vi "SUB_Read_specifFile_anyFolder.vi"(2 "name or relative path":string, 3 "Base path":string) -> (0 "error out":errorcluster, 1 "text":string)   [LabVIEW 2011]
panel:
  out "path":path
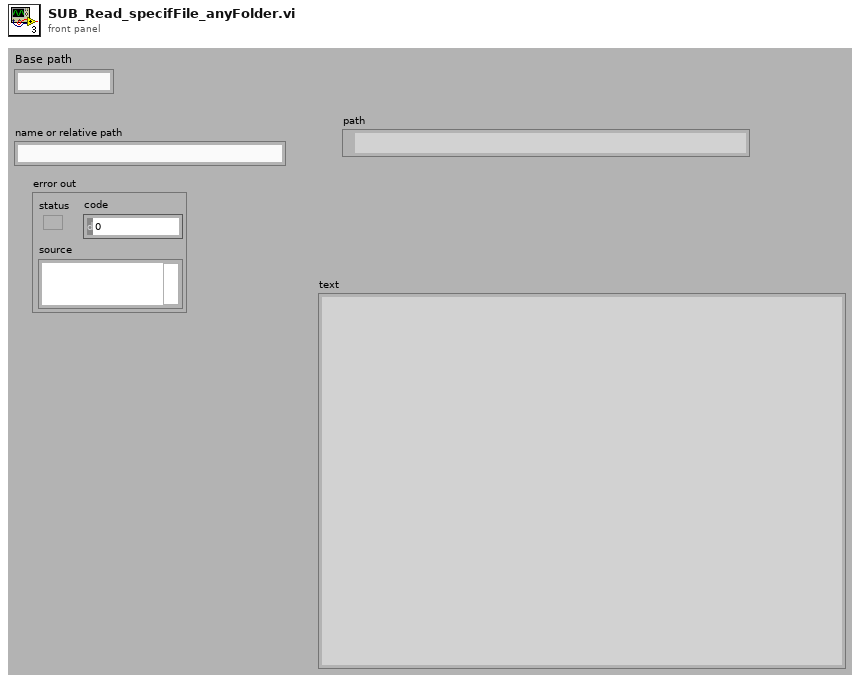
[diagram p1: front panel]
types:
  T1 = enum16{"open", "replace", "create", "open or create", "replace or create", "replace or create with confirmation"}
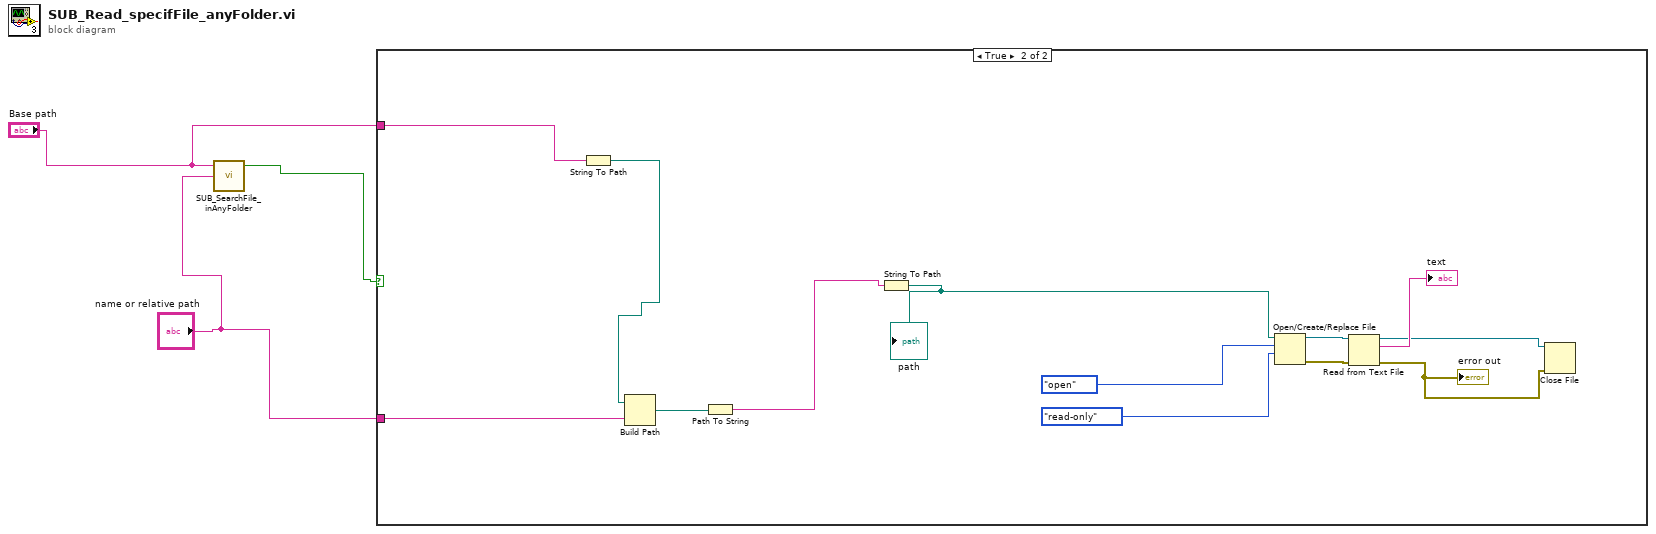
[diagram p0: block diagram]
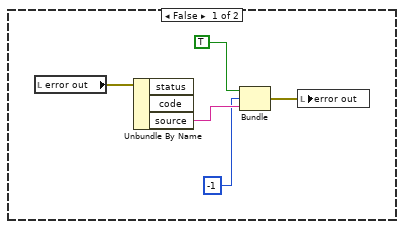
[diagram p2: hidden frame]
diagram:
  n1 = call "SUB_SearchFile_inAnyFolder.vi"("Search Filename in Folder"="name or relative path", "Base path"="Base path") -> ("File Existing True/Flase"=w1:bool)  [unwired: 1 in, 2 out]
  n2 = case shown="True" w1 {
    tunnel: "name or relative path" -> [_ w11]
    tunnel: "Base path" -> [_ w9]
    frame False {
      n3 = local read "error out"() -> (w8:errorcluster)
      n4 = Unbundle By Name(w8) -> ("source"=w7:string)  [unwired: 2 out]
      n5 = Bundle(TRUE, -1, "source"=w7) -> (w4:cluster{bool, i32, "source":string})  [unwired: 1 in]
      n6 = local write "error out"(w4) -> ()
    }
    frame True {
      n7 = String To Path(string=w9) -> (path=w10:path)
      n8 = Build Path(base path=w10, name or relative path=w11) -> (appended path=w13:path)
      n9 = Path To String(path=w13) -> (string=w12:string)
      n10 = String To Path(string=w12) -> (path=w16:path)
      "path" <- w16
      n11 = Open/Create/Replace File(file path (use dialog)=w16, operation (0:open)=T1."open", access (0:read/write)=enum16{"read/write", "read-only", "write-only"}."read-only") -> (refnum out=w19:refnum<file>, error out=w18:errorcluster)  [unwired: 3 in, 1 out]
      n12 = Read from Text File(file (use dialog)=w19, error in=w18) -> (refnum out=w15:refnum<file>, text=→"text":string, error out=w14:errorcluster)  [unwired: 2 in, 1 out]
      "error out" <- w14
      n13 = Close File(refnum=w15, error in=w14) -> ()  [unwired: 2 out]
    }
  }
